vi "NewExcelFile.vi"(8 "error in (no error)":errorcluster, 10 "worksheetName":string) -> (0 "error out":errorcluster, 3 "ExcelFile out":refnum<class "PortableExcelFileManipulationOXML.lvclass">)   [LabVIEW 2019, in "PortableExcelFileManipulationOXML.lvclass"]
doc: "Create a new excel file in memory with a spreadsheet named with the input string."
uses:
  PortableExcelFileManipulationOXML.lvclass
  H:/LV projects/ExpressionEvaluator/Excel/ExcelManipulation.dll
  ExcelManipulation.dll
  PortableExcelFileManipulationOXML.lvclass/PortableExcelFileManipulationOXML.ctl
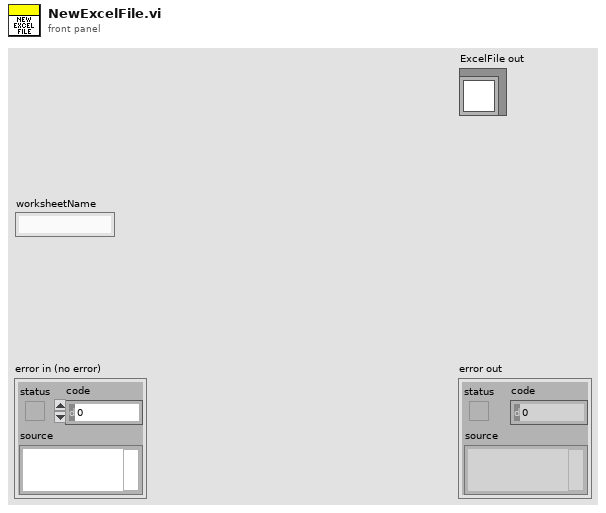
[diagram p1: front panel]
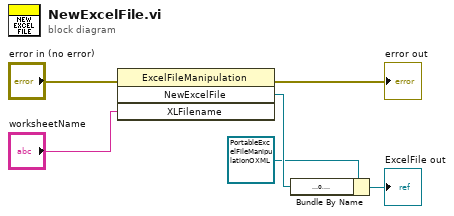
[diagram p0: block diagram]
diagram:
  n1 = invoke class="ExcelFileManipulation" method="NewExcelFile"(error in="error in (no error)", "XLFilename"="worksheetName") -> (error out=→"error out":errorcluster, "NewExcelFile"=w5:refnum<k24>)  [unwired: 2 in, 2 out]
  n2 = Bundle By Name(cluster=refnum<class "PortableExcelFileManipulationOXML.lvclass"> refnum ("ExcelFile out 2"), "ExcelOpen"=w5) -> (→"ExcelFile out":refnum<class "PortableExcelFileManipulationOXML.lvclass">)
